vi "GUARDADO.vi"() -> ()   [LabVIEW 2019]
uses:
  <vilib>/drjdpowell/SQLite Library/SQL Connection/Open (path).vi
  <vilib>/drjdpowell/SQLite Library/SQL Connection/Open (string).vi
  <vilib>/AdvancedString/Path To Command Line String.vi
  <vilib>/drjdpowell/SQLite Library/SQL Connection/Execute SQL.vi
  <vilib>/drjdpowell/SQLite Library/SQL Connection/Connection.lvclass
  <vilib>/drjdpowell/SQLite Library/SQLite.lvlib
panel:
  out "PRODUCTOS":string[][](array[string])
  in  "stop":bool
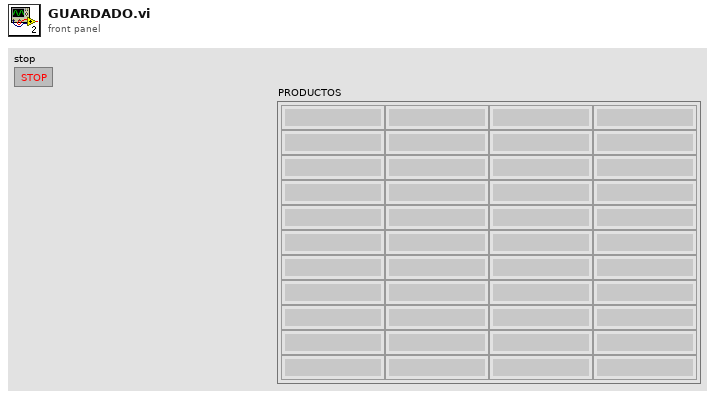
[diagram p1: front panel]
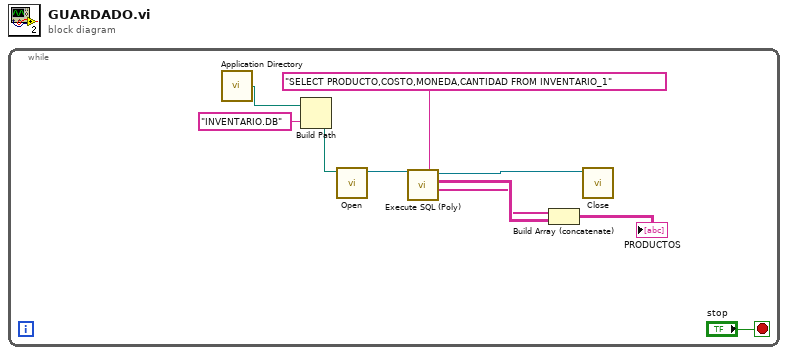
[diagram p0: block diagram]
diagram:
  n1 = while {
    stop <- "stop" stop-if-true
    n2 = call <vilib>:"Application Directory.vi"() -> ("Application Directory"=w9:path)
    n3 = Build Path(base path=w9, name or relative path="INVENTARIO.DB") -> (appended path=w7:path)
    n4 = call-poly <vilib>:"Open.vi"("db file"=w7) -> ("SQLite Connection"=w6:refnum<class "Connection.lvclass">)  [unwired: 9 in, 1 out]
    n5 = call-poly <vilib>:"Execute SQL (Poly).vi"("SQL"="SELECT PRODUCTO,COSTO,MONEDA,CANTIDAD FROM INVENTARIO_1", "SQLite Connection in"=w6) -> ("Column Names"=w2:string[], "Result Set"=w3:string[][], "SQLite Connection"=w5:refnum<class "Connection.lvclass">)  [unwired: 6 in, 1 out]
    n6 = Build Array (concatenate)(w2, w3) -> (→"PRODUCTOS":string[][])
    n7 = call-dynamic "Close.vi"("SQLite Connection in"=w5) -> ()  [unwired: 10 in, 1 out]
  }
